vi "get project directory.vi"(8 "error in (no error)":errorcluster, 11 "VI path":path) -> (0 "error out":errorcluster, 2 "already existed":bool, 3 "project directory":path)   [LabVIEW 2014, in "CD model script.lvlib"]
uses:
  CD model script.lvlib
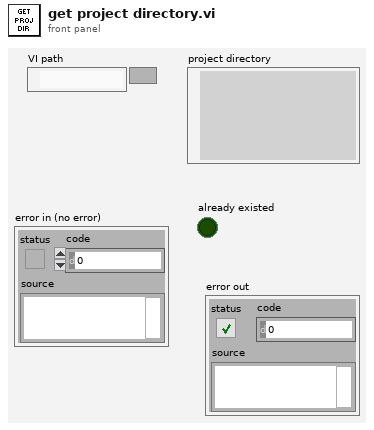
[diagram p1: front panel]
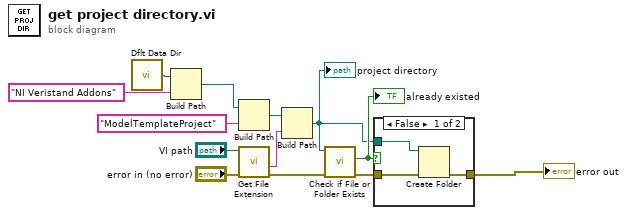
[diagram p0: block diagram]
diagram:
  n1 = call <vilib>:"Dflt Data Dir.vi"() -> ("App:Default Data Directory"=w10:path)
  n2 = Build Path(base path=w10, name or relative path="NI Veristand Addons") -> (appended path=w8:path)
  n3 = Build Path(base path=w8, name or relative path="ModelTemplateProject") -> (appended path=w11:path)
  n4 = call <vilib>:"Get File Extension.vi"("error in (no error)"="error in (no error)", "file"="VI path") -> ("error out"=w2:errorcluster, "filename without extension"=w13:string)  [unwired: 6 in, 2 out]
  n5 = Build Path(base path=w11, name or relative path=w13) -> (appended path=w5:path)
  "project directory" <- w5
  n6 = call <vilib>:"Check if File or Folder Exists.vi"("error in (no error)"=w2, "path"=w5) -> ("error out"=w4:errorcluster, "file or folder exists?"=w6:bool)  [unwired: 7 in, 1 out]
  "already existed" <- w6
  n7 = case shown="False" w6 {
    tunnel: w5 -> [w16 _]
    tunnel: w4 -> [w15 w17]
    tunnel: [w14 w17] -> w3
    frame False {
      n8 = Create Folder(path (use dialog)=w16, error in=w15) -> (error out=w14:errorcluster)  [unwired: 1 in, 2 out]
    }
    frame True {
    }
  }
  "error out" <- w3
